vi "OCR Example Tesseract.vi"() -> ()   [LabVIEW 2020, in "examples.lvlib"]
uses:
  examples.lvlib
  feature_detection/Text Tesseract/Detection Result.ctl
  feature_detection/Text Tesseract/Rectangle Corners.ctl
  common/Image Point (Integer).ctl
  image/ARGB Colour.ctl
  common/Image Size (Integer).ctl
  <vilib>/Utility/sysdir.llb/System Directory Type.ctl
  feature_detection/Text Tesseract/Text Tesseract.lvclass/Text Tesseract.ctl
  image/New Image (ARGB Preallocated).vi
  feature_detection/Text Tesseract/Run (ARGB).vi
  image/Draw Image to Picture (ARGB).vi
  image/New Image (ARGB Preallocated).vi/3321fa97-f432-4e1e-8db9-a0df79aed21b.vi
  image/ARGB Colour to U32 Pixel Value.vi
  image/Draw Text (ARGB).vi/0015c4fc-6a12-4f82-815b-6c2f827f408b.vi
  feature_detection/Text Tesseract/Run (ARGB).vi/d21e2b8c-d7dd-47ce-9b78-18a6692dbbcb.vi
  image/Draw Rectangle (ARGB).vi/7e6fb015-3761-4366-a0a7-e436eb229083.vi
  image/Draw Image to Picture (ARGB).vi/8cd07b1b-062e-4fe4-9e87-2eb3dc89fe0e.vi
  <vilib>/Utility/error.llb/Error Cluster From Error Code.vi
  image/image.lvlib
  common/common.lvlib
  feature_detection/Text Tesseract/Text Tesseract.lvclass
panel:
  in  "tessdata":path=path "" caption="Tesseract-OCR tessdata directory - leave <Not a Path> to use expected location"
  out "Detections":T1[](array[typedef])
  out "Detected Text":string
  out "Output":picture
  # "See Block Diagram for Instructions on Downloading Tesseract-OCR V5"
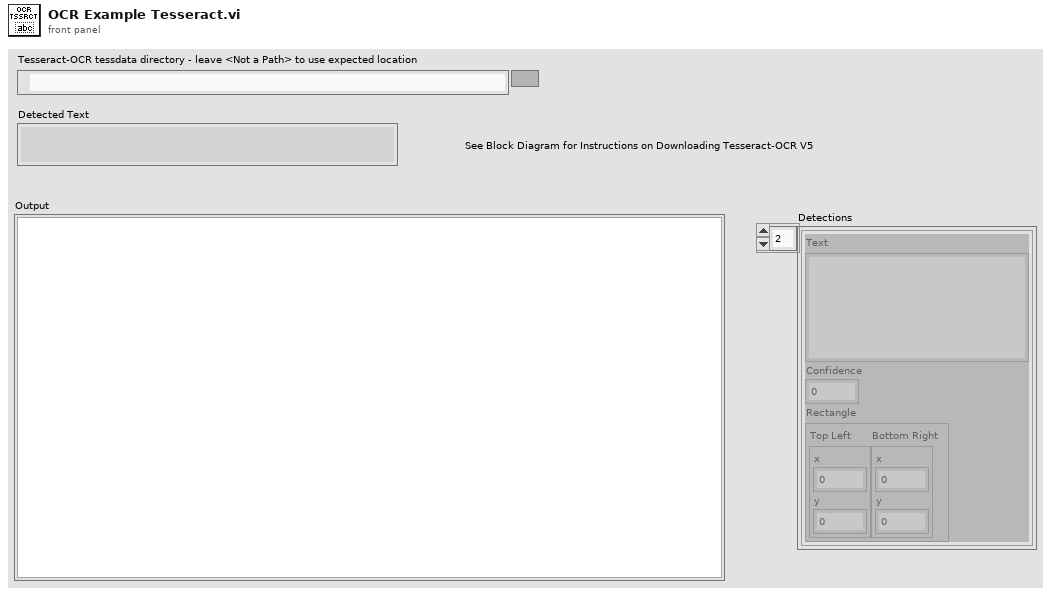
[diagram p1: front panel]
types:
  T1 = typedef "feature_detection.lvlib/Text Tesseract.lvclass/Detection Result.ctl" = cluster{"Text":string, "Confidence":sgl, "Rectangle":T2}
  T2 = typedef "feature_detection.lvlib/Text Tesseract.lvclass/Rectangle Corners.ctl" = cluster{"Top Left":T3, "Bottom Right":T3}
  T3 = typedef "common.lvlib/Image Point (Integer).ctl" = cluster{"x":i32, "y":i32}
  T4 = typedef "image.lvlib/ARGB Colour.ctl" = cluster{"Alpha":u8, "RGB":u32}
  T5 = typedef "common.lvlib/Image Size (Integer).ctl" = cluster{"Width":u16, "Height":u16}
  T6 = typedef "System Directory Type.ctl" = i32
  T7 = typedef "image.lvlib/ARGB Image.ctl" = refnum<data-value>
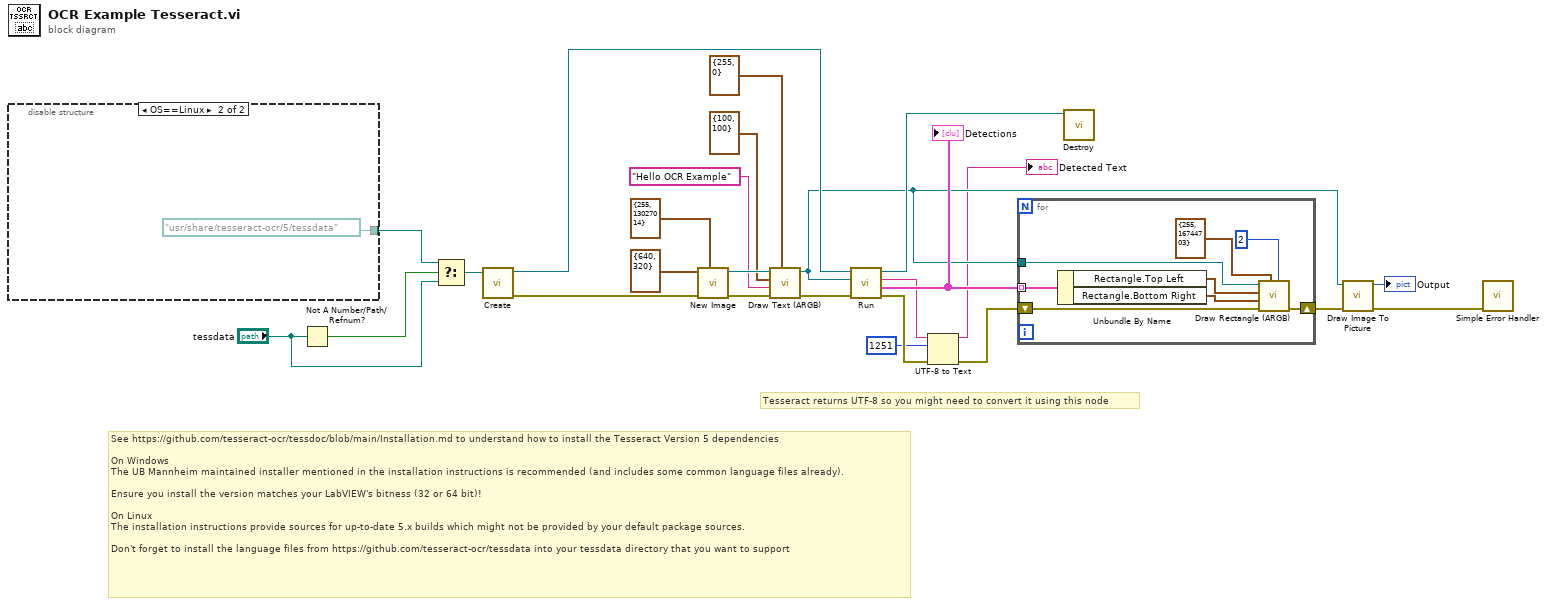
[diagram p0: block diagram]
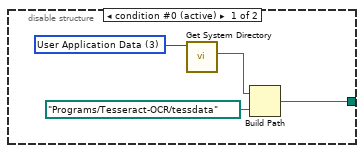
[diagram p2: hidden frame]
diagram:
  # "Tesseract returns UTF-8 so you might need to convert it using this node"
  # "See https://github.com/tesseract-ocr/tessdoc/blob/main/Installation.md to understand how to install the Tesseract Version 5 dependencies\n\nOn Windows\nThe UB Mannheim maintained installer mentioned in the installation instructions is recommended (and includes some common language files already).\n\nEnsure you install the version matches your LabVIEW's bitness (32 or 64 bit)!\n\nOn Linux \nThe installation instructions provide sources for up-to-date 5.x builds which might not be provided by your default package sources.\n\nDon't forget to install the language files from https://github.com/tesseract-ocr/tessdata into your tessdata directory that you want to support"
  n1 = disable-structure shown="OS==Linux" {
    disable-tunnel: [w26 path "/usr/share/tesseract-ocr/5/tessdata" ("appended path")] -> w8
    frame condition #0 (active) {
      w29 = T6 3 items=["User Home"=0, "User Desktop"=1, "User Documents"=2, "User Application Data"=3, "User Preferences"=4, "User Temporary"=5, "Public Documents"=6, "Public Application Data"=7, "Public Preferences"=8, "Public Cache"=13, "System Core Libraries"=9, "System Installed Libraries"=10, "Application Files"=11, "Boot Volume Root"=12] ("system directory type")
      n2 = call <vilib>:"Get System Directory.vi"("system directory type"=w29) -> ("system directory"=w28:path)  [unwired: 10 in]
      n3 = Build Path(base path=w28, name or relative path=path "Programs/Tesseract-OCR/tessdata") -> (appended path=w26:path)
    }
    frame condition #1 {
    }
  }
  n4 = Not A Number/Path/Refnum?(number/path/refnum="tessdata") -> (NaN/Path/Refnum?=w6:bool)
  n5 = Select(t=w8, s=w6, f="tessdata") -> (s? t:f=w7:path)
  n6 = call "Create.vi"("Data Path (Empty: Use System Path)"=w7) -> ("error out"=w15:errorcluster, "Text Tesseract"=w14:refnum<class "Text Tesseract.lvclass">)  [unwired: 9 in]
  n7 = call-poly "New Image.vi"("Colour (Default: Black)"=T4 {"Alpha"=255, "RGB"=13027014}, "error in (no error)"=w15, "Preallocated Image Size (Default: 0,0)"=T5 {"Width"=640, "Height"=320}) -> ("error out"=w21:errorcluster, "ARGB Image"=w22:T7)  [unwired: 7 in]
  n8 = call "Draw Text (ARGB).vi"("ARGB Colour"=T4 {"Alpha"=255, "RGB"=0}, "error in (no error)"=w21, "Text"="Hello OCR Example", "Origin"=T3 {"x"=100, "y"=100}, "ARGB Image in"=w22) -> ("error out"=w13:errorcluster, "ARGB Image"=w9:T7)  [unwired: 5 in]
  n9 = call-poly "Run.vi"("error in (no error)"=w13, "ARGB Image in"=w9, "Text Tesseract in"=w14) -> ("error out"=w25:errorcluster, "Detections"=w12:T1[], "Detected Text"=w2:string, "Text Tesseract"=w11:refnum<class "Text Tesseract.lvclass">)  [unwired: 5 in]
  "Detections" <- w12
  n10 = UTF-8 to Text(8:w25, 10:1251 ("encoding (system default=-1)"), 11:w2) -> (0:w3:errorcluster, 3:→"Detected Text":string)
  n11 = for {
    tunnel: w12 -> [w36] mode=indexing
    shift-right: [w37] -> w23
    shift-left: w3 -> [w38]
    tunnel: w9 -> [w33]
    n12 = Unbundle By Name(w36) -> ("Rectangle.Top Left"=w32:T3, "Rectangle.Bottom Right"=w31:T3)
    n13 = call "Draw Rectangle (ARGB).vi"("Thickness (Default: 1)"=2, "ARGB Colour"=T4 {"Alpha"=255, "RGB"=16744703}, "error in (no error)"=w38, "Point B"=w31, "Point A"=w32, "ARGB Image in"=w33) -> ("error out"=w37:errorcluster)  [unwired: 4 in, 1 out]
  }
  n14 = call "Destroy.vi"("Text Detector in"=w11) -> ()  [unwired: 10 in, 1 out]
  n15 = call-poly "Draw Image To Picture.vi"("error in (no error)"=w23, "ARGB Image Source in"=w9) -> ("error out"=w10:errorcluster, "Picture"=→"Output":picture)  [unwired: 8 in]
  n16 = call <vilib>:"Simple Error Handler.vi"("error in (no error)"=w10) -> ()  [unwired: 4 in, 5 out]
